vi "AIDI-Engine.vi"(0 "Config":T1, 2 "Action":T4, 11 "error in (no error)":errorcluster) -> (6 "AI":dbl[][](array[numeric]), 8 "DI":bool[][](array[boolean]), 10 "Position":dbl, 15 "error out":errorcluster)   [LabVIEW 2020]
uses:
  Typedefs/AIDI-Action.ctl
  Typedefs/AIDI-Config.ctl
  Typedefs/AIDI-Output Spec.ctl
  Typedefs/DI-Output Spec.ctl
  <resource>/objmgr/daqmx.rc
panel:
  in  "Timeout (s)":dbl format="%#_13g"
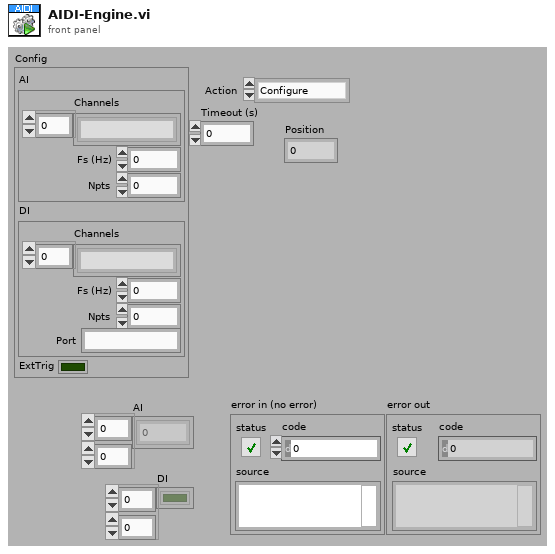
[diagram p1: front panel]
types:
  T1 = typedef "AIDI-Config.ctl" = cluster{"AI":T2, "DI":T3, "ExtTrig":bool}
  T2 = typedef "AIDI-Output Spec.ctl" = cluster{"Channels":string[], "Fs (Hz)":dbl, "Npts":i32}
  T3 = typedef "DI-Output Spec.ctl" = cluster{"Channels":string[], "Fs (Hz)":dbl, "Npts":i32, "Port":string}
  T4 = typedef "AIDI-Action.ctl" = enum16{"Configure", "Initialize", "Start", "Read", "Clean up", "Init & Start", "Config & Test", "Position"}
  T5 = typedef "AIDI-Task Specification.ctl" = cluster{"Task":refnum<k21>, "Channels":string, "Dual channel":bool, "Index":i32[]}
  T6 = typedef "AIDI-DI Tasks.ctl" = cluster{"Active":bool, "DI task":refnum<k21>}
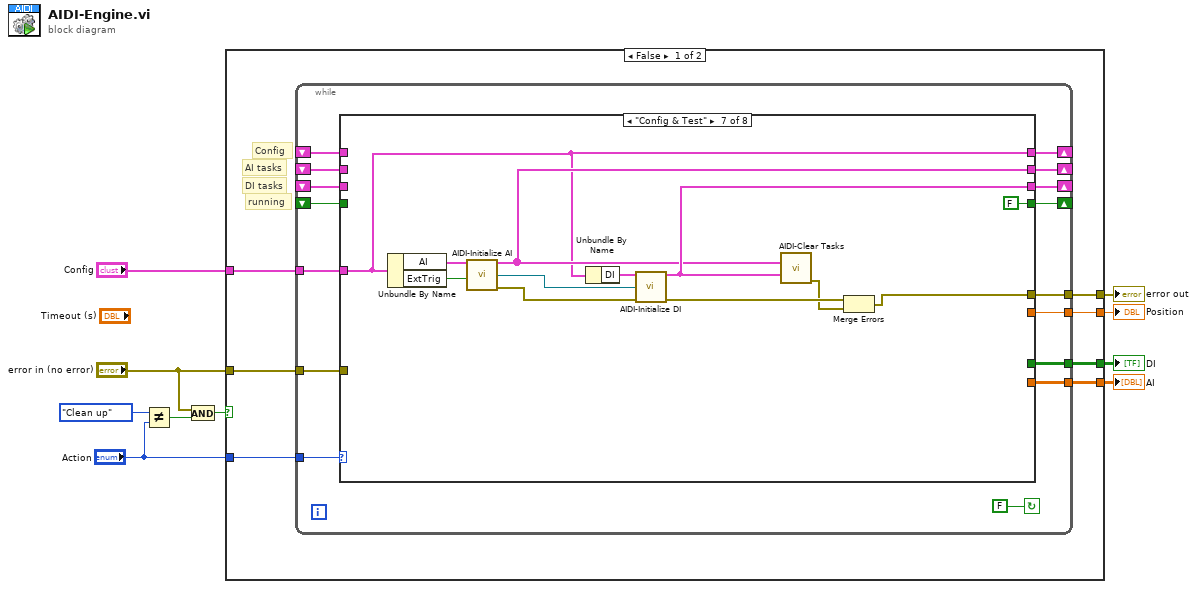
[diagram p0: block diagram]
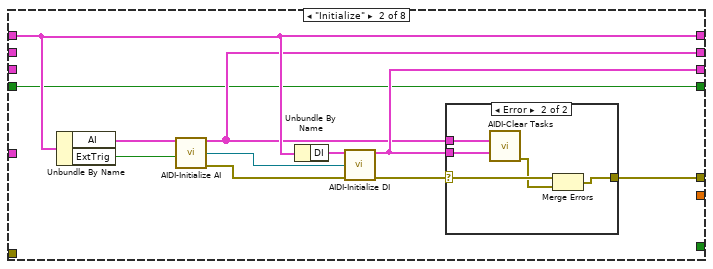
[diagram p3: hidden frame]
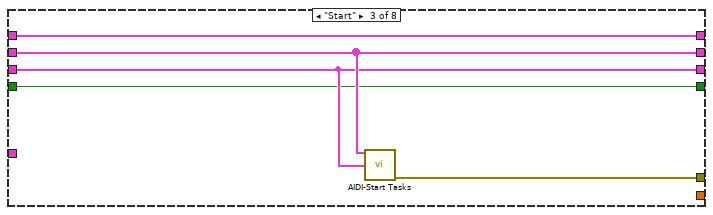
[diagram p5: hidden frame]
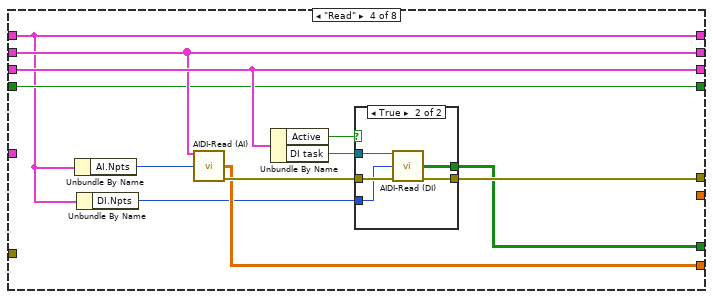
[diagram p6: hidden frame]
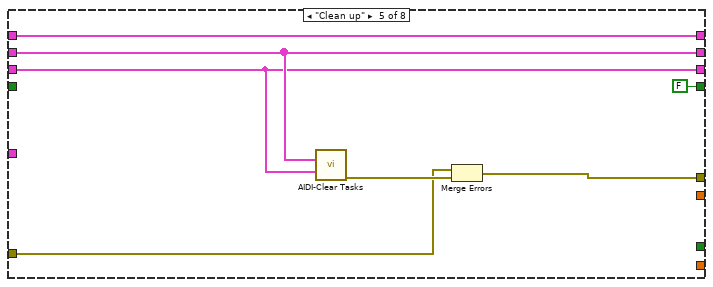
[diagram p8: hidden frame]
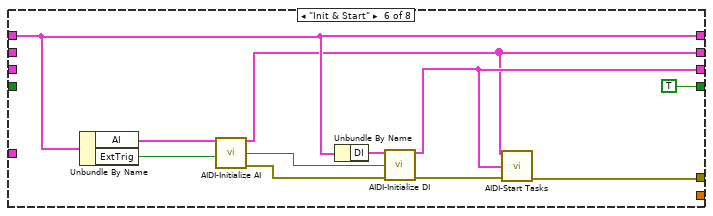
[diagram p9: hidden frame]
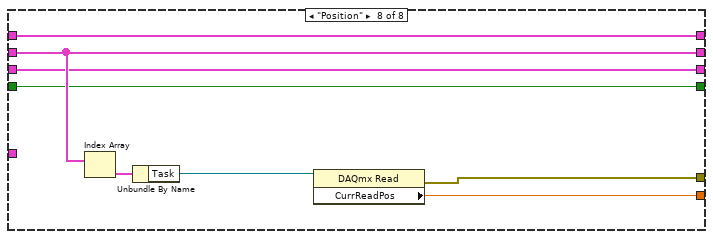
[diagram p10: hidden frame]
diagram:
  n1 = Not Equal?(x=AIDI-Action."Clean up", y="Action") -> (x != y?=w5:bool)
  n2 = And(x="error in (no error)", y=w5) -> (x .and. y?=w6:bool)
  n3 = case shown="False" w6 {
    tunnel: "Action" -> [w17 _]
    tunnel: [w16 w115] -> w10
    tunnel: "Config" -> [w15 _]
    tunnel: "error in (no error)" -> [w11 w115]
    tunnel: [w14 _] -> w3
    tunnel: [w13 _] -> w2
    tunnel: [w12 _] -> w1
    frame False {
      # "running"
      # "Config"
      # "DI tasks"
      # "AI tasks"
      n4 = while {
        shift-right: [w25] -> _
        shift-left: _ -> [w32]
        shift-right: [w31] -> _
        shift-left: _ -> [w30]
        tunnel: [w29] -> w16
        tunnel: w15 -> [w27]
        shift-right: [w28] -> _
        shift-left: _ -> [w26]
        tunnel: w17 -> [w33]
        tunnel: [w23] -> w14
        shift-right: [w22] -> _
        shift-left: _ -> [w21]
        tunnel: [w20] -> w13
        tunnel: [w19] -> w12
        tunnel: w11 -> [w18]
        stop <- FALSE continue-if-true
        n5 = case shown="\"Config & Test\"" w33 {
          tunnel: [_ w40 w55 w64 w78 w86 w99 w110] -> w29
          tunnel: w32 -> [w36 _ w57 w66 w82 _ _ w113]
          tunnel: [w35 w42 w56 w70 w80 w88 w101 w107] -> w31
          tunnel: w30 -> [w35 _ w56 w70 w80 _ _ w107]
          tunnel: [w37 w44 w58 w60 w81 w90 w97 w114] -> w28
          tunnel: w27 -> [w37 _ _ _ _ _ w97 _]
          tunnel: w26 -> [_ w44 w58 w60 w81 w90 _ w114]
          tunnel: [w36 w41 w57 w66 w82 w87 w100 w113] -> w25
          tunnel: [_ _ _ _ _ _ _ w111] -> w23
          tunnel: [w34 w39 w54 w65 FALSE TRUE FALSE w108] -> w22
          tunnel: w21 -> [w34 w39 w54 w65 _ _ _ w108]
          tunnel: [_ _ _ w63 _ _ _ _] -> w20
          tunnel: [_ _ _ w62 _ _ _ _] -> w19
          tunnel: w18 -> [_ _ _ _ w77 _ _ _]
          frame "Configure", Default {
          }
          frame "Initialize" {
            n6 = Unbundle By Name(w44) -> ("AI"=w48:T2, "ExtTrig"=w38:bool)
            n7 = call "AIDI-Initialize AI.vi"("AI"=w48, "external trig"=w38) -> ("Tasks Out"=w41:T5[], "Sync Task"=w45:refnum<k21>, "error out"=w47:errorcluster)  [unwired: 11 in]
            n8 = Unbundle By Name(w44) -> ("DI"=w46:T3)
            n9 = call "AIDI-Initialize DI.vi"("DI"=w46, "Sync Task"=w45, "error in (no error)"=w47) -> ("DI Tasks"=w42:T6, "error out"=w43:errorcluster)  [unwired: 11 in]
            n10 = case shown="Error" w43 {
              selector: w43 -> [_ w52]
              tunnel: w42 -> [_ w49]
              tunnel: w41 -> [_ w53]
              tunnel: [_ w50] -> w40
              frame No Error {
              }
              frame Error {
                n11 = call "AIDI-Clear Tasks.vi"("AI Tasks"=w53, "DI Tasks"=w49) -> ("error out"=w51:errorcluster)  [unwired: 13 in]
                n12 = Merge Errors(w52, w51) -> (w50:errorcluster)
              }
            }
          }
          frame "Start" {
            n13 = call "AIDI-Start Tasks.vi"("AO Tasks"=w57, "DO Tasks"=w56) -> ("error out"=w55:errorcluster)  [unwired: 13 in]
          }
          frame "Read" {
            n14 = Unbundle By Name(w60) -> ("AI.Npts"=w61:i32)
            n15 = Unbundle By Name(w60) -> ("DI.Npts"=w59:i32)
            n16 = call "AIDI-Read (AI).vi"("Tasks In"=w66, "number of samples per channel"=w61) -> ("AO Waveforms"=w63:dbl[][], "error out"=w68:errorcluster)  [unwired: 11 in, 1 out]
            n17 = Unbundle By Name(w70) -> ("Active"=w69:bool, "DI task"=w67:refnum<k21>)
            n18 = case shown="True" w69 {
              tunnel: w68 -> [w71 w75]
              tunnel: w67 -> [_ w76]
              tunnel: [w71 w74] -> w64
              tunnel: [_ w73] -> w62
              tunnel: w59 -> [_ w72]
              frame False {
              }
              frame True {
                n19 = call "AIDI-Read (DI).vi"("Task In"=w76, "number of samples per channel"=w72, "error in (no error)"=w75) -> ("DO Waveforms"=w73:bool[][], "error out"=w74:errorcluster)  [unwired: 10 in, 1 out]
              }
            }
          }
          frame "Clean up" {
            n20 = call "AIDI-Clear Tasks.vi"("AI Tasks"=w82, "DI Tasks"=w80) -> ("error out"=w83:errorcluster)  [unwired: 13 in]
            n21 = Merge Errors(w77, w83) -> (w78:errorcluster)
          }
          frame "Init & Start" {
            n22 = Unbundle By Name(w90) -> ("AI"=w94:T2, "ExtTrig"=w84:bool)
            n23 = call "AIDI-Initialize AI.vi"("AI"=w94, "external trig"=w84) -> ("Tasks Out"=w87:T5[], "Sync Task"=w91:refnum<k21>, "error out"=w93:errorcluster)  [unwired: 11 in]
            n24 = Unbundle By Name(w90) -> ("DI"=w92:T3)
            n25 = call "AIDI-Initialize DI.vi"("DI"=w92, "Sync Task"=w91, "error in (no error)"=w93) -> ("DI Tasks"=w88:T6, "error out"=w89:errorcluster)  [unwired: 11 in]
            n26 = call "AIDI-Start Tasks.vi"("AO Tasks"=w87, "DO Tasks"=w88, "error in (no error)"=w89) -> ("error out"=w86:errorcluster)  [unwired: 12 in]
          }
          frame "Config & Test" {
            n27 = Unbundle By Name(w97) -> ("AI"=w106:T2, "ExtTrig"=w95:bool)
            n28 = call "AIDI-Initialize AI.vi"("AI"=w106, "external trig"=w95) -> ("Tasks Out"=w100:T5[], "Sync Task"=w103:refnum<k21>, "error out"=w105:errorcluster)  [unwired: 11 in]
            n29 = Unbundle By Name(w97) -> ("DI"=w104:T3)
            n30 = call "AIDI-Initialize DI.vi"("DI"=w104, "Sync Task"=w103, "error in (no error)"=w105) -> ("DI Tasks"=w101:T6, "error out"=w102:errorcluster)  [unwired: 11 in]
            n31 = call "AIDI-Clear Tasks.vi"("AI Tasks"=w100, "DI Tasks"=w101) -> ("error out"=w98:errorcluster)  [unwired: 13 in]
            n32 = Merge Errors(w102, w98) -> (w99:errorcluster)
          }
          frame "Position" {
            n33 = Index Array(array=w113) -> (element=w112:T5)  [unwired: 1 in]
            n34 = Unbundle By Name(w112) -> ("Task"=w109:refnum<k21>)
            n35 = property class="DAQmx Read"(reference=w109) -> (error out=w110:errorcluster, "CurrReadPos"=w111:dbl)  [unwired: 1 in, 1 out]
          }
        }
      }
    }
    frame True {
    }
  }
  "AI" <- w2
  "DI" <- w1
  "error out" <- w10
  "Position" <- w3
